vi "Actor Core.vi"(8 "error in":errorcluster, 11 "BasicChartBinding In":refnum<class "BasicChartBinding.lvclass">) -> (0 "error out":errorcluster, 3 "Actor out":refnum<class "Actor.lvclass">)   [LabVIEW 2018, in "TestViewables.lvlib" / "BasicChartBinding.lvclass"]
doc: "(<B>Filename</B>: Actor Framework.lvlib:Actor.lvclass:Actor Core.vi)\n\nReceives messages to the actor, reacts to them, and initiates any error handling that may shut the actor down.\n\nDescendant classes may override this VI to append parallel tasks for the actor to complete while it handles messages. Overrides use the Call Parent Method node.\n\n<License>\nCopyright © 2017 Composed Systems, LLC | All rights reserved\nwww.composed.io\n\nAuthor: Ethan Stern <ethan.stern@composed.io>\n\nThis software is provided \"AS IS\" WITHOUT WARRANTIES, either express or implied, AND IS FOR EDUCATIONAL PURPOSES ONLY.\n</License>"
uses:
  BasicChartBinding.lvclass
  modules/mva-viewable/Source/IViewable/IViewable/IViewable.lvclass
  <vilib>/ActorFramework/Actor/Actor.lvclass
panel:
  out "Random Number":dbl(graph)
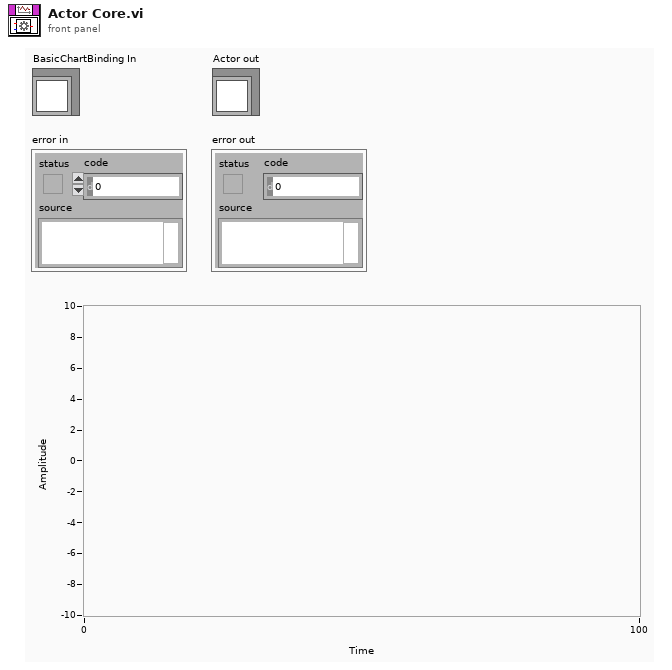
[diagram p1: front panel]
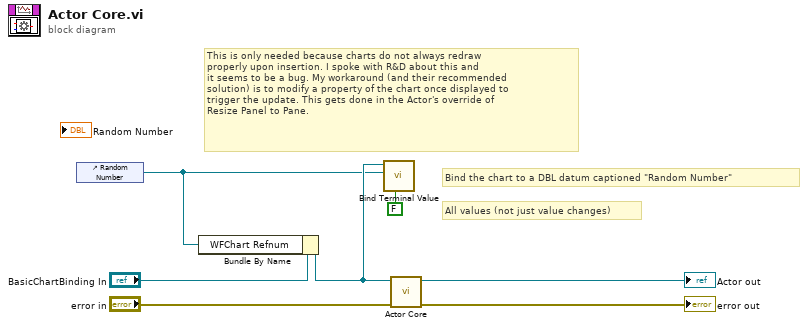
[diagram p0: block diagram]
diagram:
  # "This is only needed because charts do not always redraw\nproperly upon insertion. I spoke with R&D about this and\nit seems to be a bug. My workaround (and their recommended\nsolution) is to modify a property of the chart once displayed to\ntrigger the update. This gets done in the Actor's override of\nResize Panel to Pane."
  # "All values (not just value changes)"
  # "Bind the chart to a DBL datum captioned \"Random Number\""
  n1 = control-ref of="Random Number"() -> (w1:refnum<vi>)
  n2 = Bundle By Name(cluster="BasicChartBinding In", "WFChart Refnum"=w1) -> (w2:refnum<class "BasicChartBinding.lvclass">)
  n3 = call "Bind Terminal Value.vi"("Value Changes Only? (T)"=FALSE, "Ctl Refnum"=w1, "IViewable in"=w2) -> ()  [unwired: 7 in, 2 out]
  n4 = call-parent "Actor Core.vi"("error in"="error in", "IViewable In"=w2) -> ("error out"=→"error out":errorcluster, "Actor out"=→"Actor out":refnum<class "Actor.lvclass">)  [unwired: 8 in]
